vi "xyz-express.vi"(0 "Image":dbl[][](array[numeric]), 1 "FFT":T2, 3 "Sizes":T1, 5 "R":dbl, 9 "Threshold type":u16(ring) items=["Top fraction", "Top value"], 11 "Threshold":dbl=2.0, 12 "FFT allocated?":bool=TRUE) -> (4 "XYZ":dbl[](array[numeric]), 6 "G":dbl[][](graph), 8 "Gx":dbl[][](graph), 10 "Gy":dbl[][](graph), 15 "Filtered G":dbl[][](graph))   [LabVIEW 2015]
doc: "Single vi for calculating XYZ position of the particle.\n\nINPUT\nImage - input image\nR - radius of the window (should be >0.5)\nThreshold type, - type of threshold to apply:\n \"Top fraction\" - sets threshold as max_intensity/Threshold, e.g., for a Threshold=2 the threshold will be set to half the maximum pixel value \n \"Top value\" - sets the threshold to Threshold\nThreshold - threshold value\nFFT allocated? - must be set to true (default) if FFT and Sizes are connected. If set to False, FFT and Sizes inputs are ignored\nFFT, Sizes - Fourier transforms and sizes obtained from Local gradient preallocation\n\nOUTPUT\nXYZ - x,y position of the particle in pixels (for original image), z-value\nFiltered G - filtered local gradient magnitude image\nAuthor: Anatolii Kashchuk"
uses:
  z-split sum difference.vi
  lstsqr_lines.vi
panel:
  in  "Weights type":u16(ring)=1 items=["None", "G", "G^2"]
  # "Author: Anatolii Kashchuk"
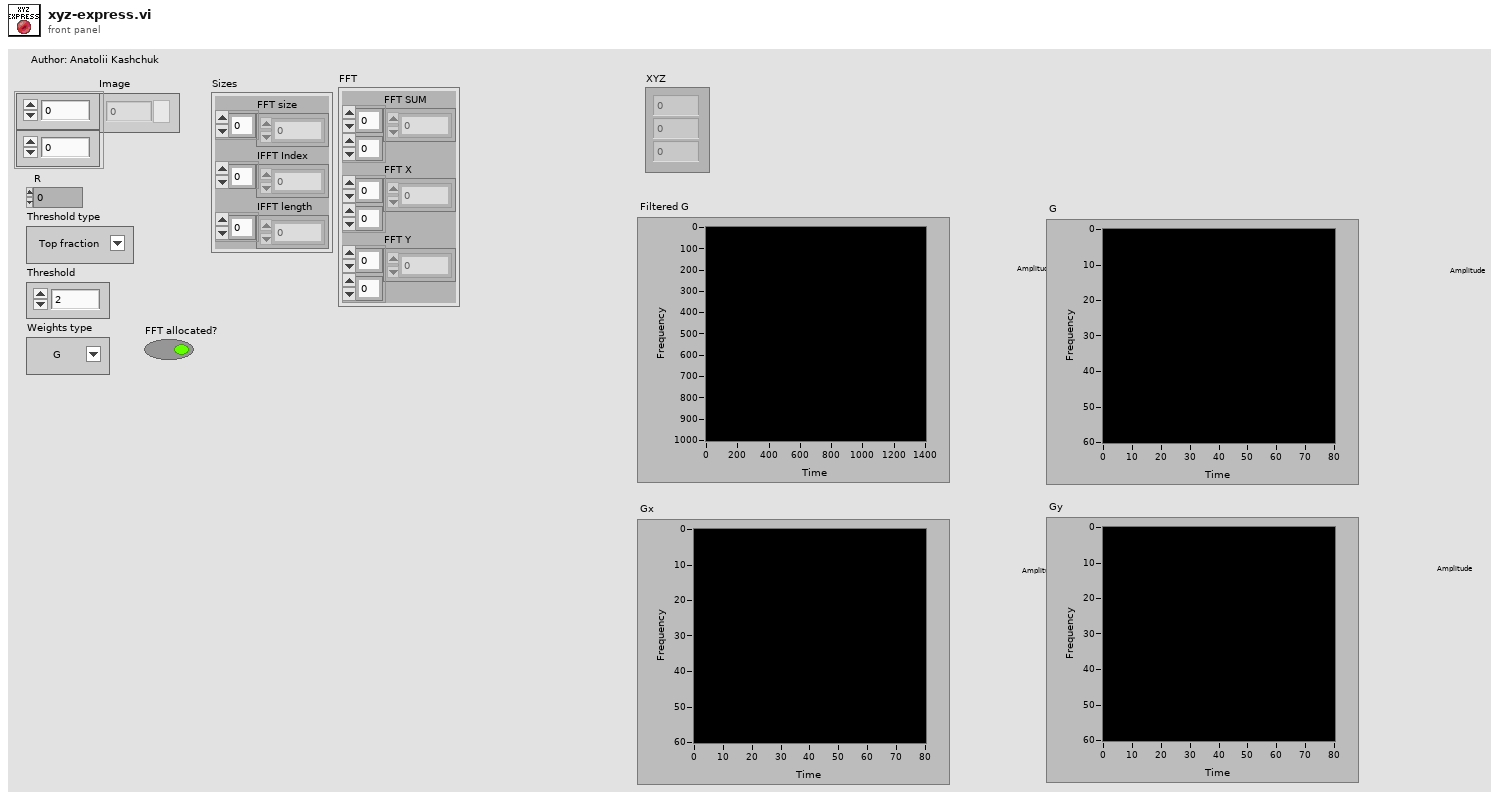
[diagram p1: front panel]
types:
  T1 = cluster{"FFT size":u32[], "IFFT Index":i32[], "IFFT length":u32[]}
  T2 = cluster{"FFT SUM":cdb[][], "FFT X":cdb[][], "FFT Y":cdb[][]}
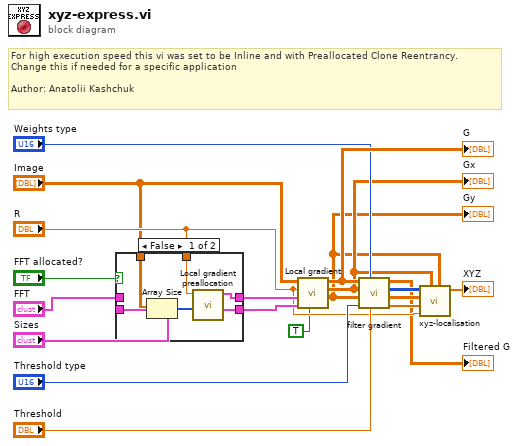
[diagram p0: block diagram]
diagram:
  # "For high execution speed this vi was set to be Inline and with Preallocated Clone Reentrancy. \nChange this if needed for a specific application\n\nAuthor: Anatolii Kashchuk"
  n1 = case shown="False" "FFT allocated?" {
    tunnel: [w24 w26] -> w16
    tunnel: [w23 w25] -> w15
    tunnel: "FFT" -> [_ w26]
    tunnel: "Sizes" -> [_ w25]
    tunnel: "R" -> [w22 _]
    tunnel: "Image" -> [w20 _]
    frame False {
      n2 = Array Size(array=w20) -> (size(s)=w21:i32[])
      n3 = call "Local gradient preallocation.vi"("Image size"=w21, "R"=w22) -> ("Sizes"=w23:T1, "FFT"=w24:T2)  [unwired: 8 in]
    }
    frame True {
    }
  }
  n4 = call "Local gradient.vi"("FFT allocated?"=TRUE, "Sizes"=w15, "FFT"=w16, "R"="R", "Image"="Image") -> ("Gy"=w7:dbl[][], "Gx"=w8:dbl[][], "G"=w19:dbl[][])  [unwired: 4 in]
  "G" <- w19
  "Gx" <- w8
  "Gy" <- w7
  n5 = call "filter gradient.vi"("Threshold"="Threshold", "Weights type"="Weights type", "Threshold type"="Threshold type", "Gy"=w7, "Gx"=w8, "G"=w19) -> ("Weights"=w9:dbl[], "gradients"=w10:dbl[][], "centers"=w11:i32[][], "Filtered G"=→"Filtered G":dbl[][])  [unwired: 2 out]
  n6 = call "xyz-localisation.vi"("Gy"=w7, "Gx"=w8, "R"="R", "weights"=w9, "B points"=w10, "A points"=w11) -> ("XYZ"=→"XYZ":dbl[])  [unwired: 5 in]
